vi "Agilent VNA Initialize.vi"(8 "error in (no error)":errorcluster, 11 "Configuration":T2={"BusType"=enum."GPIB", "GPIB Bus"=0, "GPIB Address"=16, "IP"=0, "COM"=1, "Baud Rate"=enum."9600", "USB Device"=0, "Instrument S\\N"="", "SCIL Address"=16} {"USB Device" max=31 step=1}) -> (0 "error out":errorcluster {"code" format="%.0x"}, 1 "VISA":string, 3 "dup VISA Resource Name":refnum<visa-resource-name>, 5 "Agilent VNA":T1)   [LabVIEW 2011]
uses:
  VNA Configuration.ctl
  TypeDefs/Agilent VNA Instrument Info.ctl
  TypeDefs/Agilent VNA Error Message Mode.ctl
  TypeDefs/Agilent VNA Instrument Mode.ctl
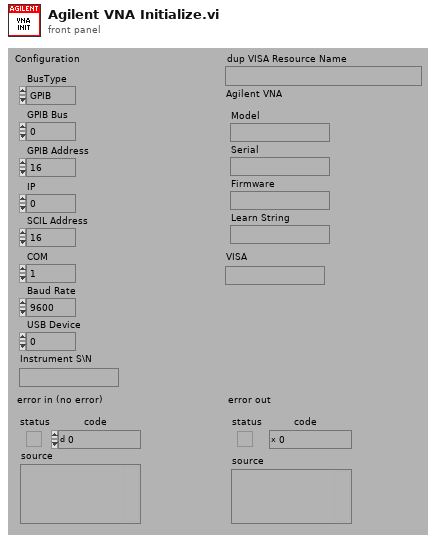
[diagram p1: front panel]
types:
  T1 = typedef "Agilent VNA Instrument Info.ctl" = cluster{"Model":string, "Serial":string, "Firmware":string, "Learn String":string}
  T2 = typedef "VNA Configuration.ctl" = cluster{"BusType":enum32{"GPIB", "LAN/IP", "Serial", "USB"}, "GPIB Bus":i32, "GPIB Address":i32, "IP":u32, "COM":i32, "Baud Rate":enum32{"300", "600", "1200", "2400", "4800", "9600"}, "USB Device":u32, "Instrument S\\N":string, "SCIL Address":i32}
  T3 = typedef "Agilent VNA Instrument Mode.ctl" = enum16{"CAT", "NA", "SA", "Power Meter", "VVM"}
  T4 = typedef "Agilent VNA Error Message Mode.ctl" = enum16{"On", "Off"}
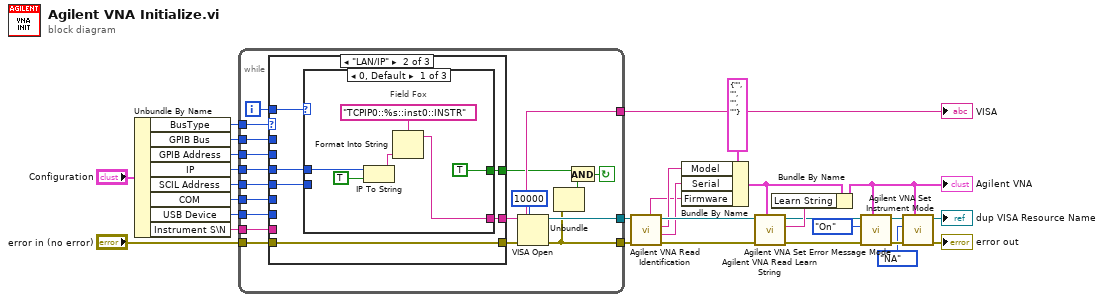
[diagram p0: block diagram]
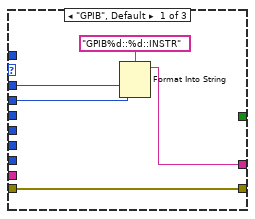
[diagram p2: hidden frame]
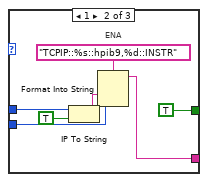
[diagram p3: hidden frame]
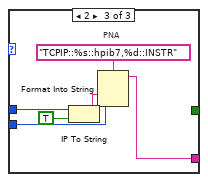
[diagram p4: hidden frame]
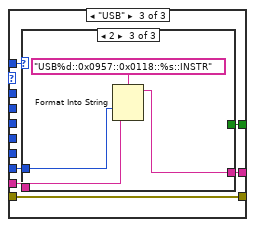
[diagram p5: hidden frame]
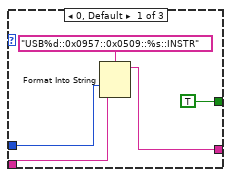
[diagram p6: hidden frame]
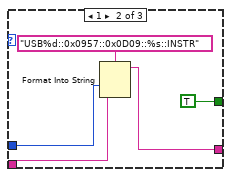
[diagram p7: hidden frame]
diagram:
  n1 = Unbundle By Name("Configuration") -> ("BusType"=w15:enum32{"GPIB", "LAN/IP", "Serial", "USB"}, "GPIB Bus"=w14:i32, "GPIB Address"=w13:i32, "IP"=w12:u32, "SCIL Address"=w11:i32, "COM"=w10:i32, "USB Device"=w9:u32, "Instrument S\\N"=w8:string)
  n2 = while {
    tunnel: "error in (no error)" -> [w48]
    tunnel: [w43] -> w20
    tunnel: [w47] -> w19
    tunnel: [w44] -> w21
    tunnel: w15 -> [w38]
    tunnel: w14 -> [w37]
    tunnel: w13 -> [w36]
    tunnel: w12 -> [w35]
    tunnel: w11 -> [w34]
    tunnel: w10 -> [w33]
    tunnel: w9 -> [w32]
    tunnel: w8 -> [w31]
    i -> [w39]
    stop <- w40 continue-if-true
    n3 = case shown="\"LAN/IP\"" w38 {
      tunnel: w48 -> [w50 w58 w83]
      tunnel: w37 -> [w53 _ _]
      tunnel: w36 -> [w52 _ _]
      tunnel: [w49 w57 w82] -> w44
      tunnel: [w50 w58 w83] -> w45
      tunnel: w33 -> [_ _ _]
      tunnel: w35 -> [_ w59 _]
      tunnel: w32 -> [_ _ w84]
      tunnel: w31 -> [_ _ w81]
      tunnel: [_ w55 w79] -> w41
      tunnel: w39 -> [_ w56 w80]
      tunnel: w34 -> [_ w54 _]
      frame "GPIB", Default {
        n4 = Format Into String(format string="GPIB%d::%d::INSTR", w53, w52) -> (resulting string=w49:string)  [unwired: 2 in, 1 out]
      }
      frame "LAN/IP" {
        n5 = case shown="0, Default" w56 {
          tunnel: w59 -> [w63 w70 w76]
          tunnel: [w62 w69 w75] -> w57
          tunnel: [TRUE ("dot notation? (F)") TRUE ("dot notation? (F)") _] -> w55
          tunnel: w54 -> [_ w66 w73]
          frame 0, Default {
            # "Field Fox"
            n6 = IP To String(1:TRUE ("dot notation? (F)"), 2:w63) -> (0:w61:string)
            n7 = Format Into String(format string="TCPIP0::%s::inst0::INSTR", w61) -> (resulting string=w62:string)  [unwired: 2 in, 1 out]
          }
          frame 1 {
            # "ENA"
            n8 = IP To String(1:TRUE ("dot notation? (F)"), 2:w70) -> (0:w68:string)
            n9 = Format Into String(format string="TCPIP::%s::hpib9,%d::INSTR", w68, w66) -> (resulting string=w69:string)  [unwired: 2 in, 1 out]
          }
          frame 2 {
            # "PNA"
            n10 = IP To String(1:TRUE ("dot notation? (F)"), 2:w76) -> (0:w74:string)
            n11 = Format Into String(format string="TCPIP::%s::hpib7,%d::INSTR", w74, w73) -> (resulting string=w75:string)  [unwired: 2 in, 1 out]
          }
        }
      }
      frame "USB" {
        n12 = case shown="2" w80 {
          tunnel: w84 -> [w88 w93 w97]
          tunnel: [w87 w92 w96] -> w82
          tunnel: w81 -> [w86 w91 w95]
          tunnel: [TRUE ("dot notation? (F)") TRUE ("dot notation? (F)") _] -> w79
          frame 0, Default {
            n13 = Format Into String(format string="USB%d::0x0957::0x0509::%s::INSTR", w88, w86) -> (resulting string=w87:string)  [unwired: 2 in, 1 out]
          }
          frame 1 {
            n14 = Format Into String(format string="USB%d::0x0957::0x0D09::%s::INSTR", w93, w91) -> (resulting string=w92:string)  [unwired: 2 in, 1 out]
          }
          frame 2 {
            n15 = Format Into String(format string="USB%d::0x0957::0x0118::%s::INSTR", w97, w95) -> (resulting string=w96:string)  [unwired: 2 in, 1 out]
          }
        }
      }
    }
    n16 = VISA Open(timeout (0)=u32 10000 ("VISA Open timeout (0)"), error in (no error)=w45, VISA resource name=w44) -> (VISA resource name=w47:refnum<visa-resource-name>, error out=w43:errorcluster)  [unwired: 2 out]
    n17 = Unbundle(w43) -> ("status"=w42:bool)  [unwired: 2 out]
    n18 = And(x=w41, y=w42) -> (x .and. y?=w40:bool)
  }
  "VISA" <- w21
  n19 = call "Agilent VNA Read Identification.vi"("error in (no error)"=w20, "VISA Resource Name"=w19) -> ("error out"=w27:errorcluster, "Serial Number"=w25:string, "Model Number"=w24:string, "dup VISA Resource Name"=w26:refnum<visa-resource-name>, "Firmware"=w23:string)  [unwired: 5 out]
  n20 = Bundle By Name(cluster=T1 {"Model"="", "Serial"="", "Firmware"="", "Learn String"=""} ("Agilent VNA"), "Model"=w24, "Serial"=w25, "Firmware"=w23) -> (w28:T1)
  n21 = call "Agilent VNA Read Learn String.vi"("Agilent VNA"=w28, "error in (no error)"=w27, "VISA Resource Name"=w26) -> ("error out"=w17:errorcluster, "Learn String"=w29:string, "dup VISA Resource Name"=w18:refnum<visa-resource-name>)  [unwired: 6 out]
  n22 = Bundle By Name(cluster=w28, "Learn String"=w29) -> (w2:T1)
  "Agilent VNA" <- w2
  n23 = call "Agilent VNA Set Error Message Mode.vi"("Agilent VNA"=w2, "error in (no error)"=w17, "Error Message Mode"=Agilent_VNA_Error_Message_Mode."On", "VISA Resource Name"=w18) -> ("error out"=w6:errorcluster, "dup VISA Resource Name"=w5:refnum<visa-resource-name>)  [unwired: 6 out]
  n24 = call "Agilent VNA Set Instrument Mode.vi"("Agilent VNA"=w2, "error in (no error)"=w6, "Instrument Mode"=Agilent_VNA_Instrument_Mode."NA", "VISA Resource Name"=w5) -> ("error out"=→"error out":errorcluster, "dup VISA Resource Name"=→"dup VISA Resource Name":refnum<visa-resource-name>)  [unwired: 6 in]
